vi "Read Recipes.vi"(8 "error in (no error)":errorcluster, 11 "Master in":refnum<class "Master.lvclass">) -> (0 "error out":errorcluster, 3 "Master out":refnum<class "Master.lvclass">)   [LabVIEW 2014, in "Master.lvclass"]
uses:
  Master/Master.lvclass
  Master/Master.lvclass/Master.ctl
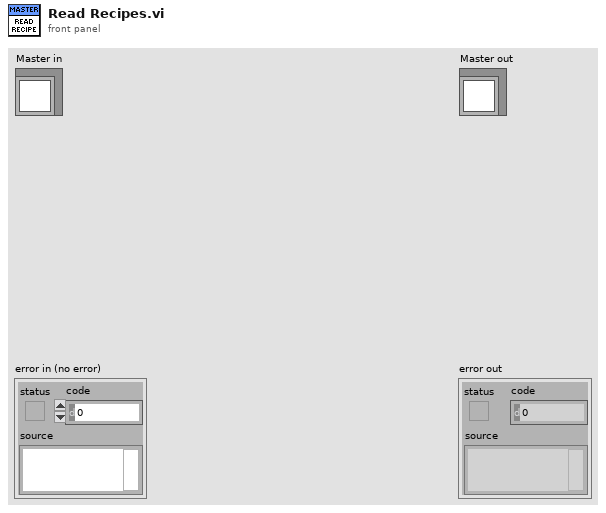
[diagram p1: front panel]
types:
  T1 = cluster{cluster{string, string, string, string, string, string}[]}
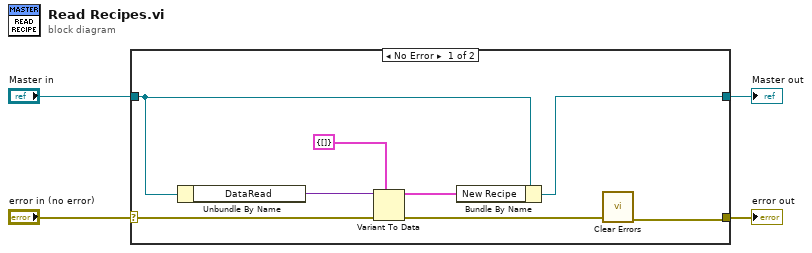
[diagram p0: block diagram]
diagram:
  n1 = case shown="No Error" "error in (no error)" {
    selector: "error in (no error)" -> [w9 w14]
    tunnel: [w5 w14] -> w3
    tunnel: [w10 w13] -> w1
    tunnel: "Master in" -> [w11 w13]
    frame No Error {
      n2 = Unbundle By Name(w11) -> ("DataRead"=w12:variant)
      n3 = Variant To Data(error in=w9, type=T1 {[]}, Variant=w12) -> (data=w8:T1, error out=w6:errorcluster)
      n4 = Bundle By Name(cluster=w11, "New Recipe"=w8) -> (w10:refnum<class "Master.lvclass">)
      n5 = call <vilib>:"Clear Errors.vi"("error in (no error)"=w6) -> ("error out"=w5:errorcluster)  [unwired: 5 in, 1 out]
    }
    frame Error {
    }
  }
  "error out" <- w3
  "Master out" <- w1
